vi "AuMT8852B Tester RS232 Baud Rate.vi"(5 "Baud Rate (1200)":T1(ring), 7 "Set/Get (Set)":enum16{"Set", "Get"}(ring), 8 "error in (no error)":errorcluster, 11 "VISA session":refnum<visa-resource-name>) -> (0 "error out":errorcluster, 2 "error code":i32, 3 "VISA session out":refnum<visa-resource-name>, 4 "Baud Rate Out":T1(ring))   [LabVIEW 2017]
doc: "Anritsu MT8852B Bluetooth Tester\n\nINPUTS\nSet/Get - whether the value is being sent to or retrieved from the instrument.\nBaud Rate - information to send to the instrument.\n\nOUTPUTS\nBaud Rate out - the present value in the instrument."
uses:
  <instrlib>/aumt8852B/General/Utilities/MT8850 Attribute ID.ctl
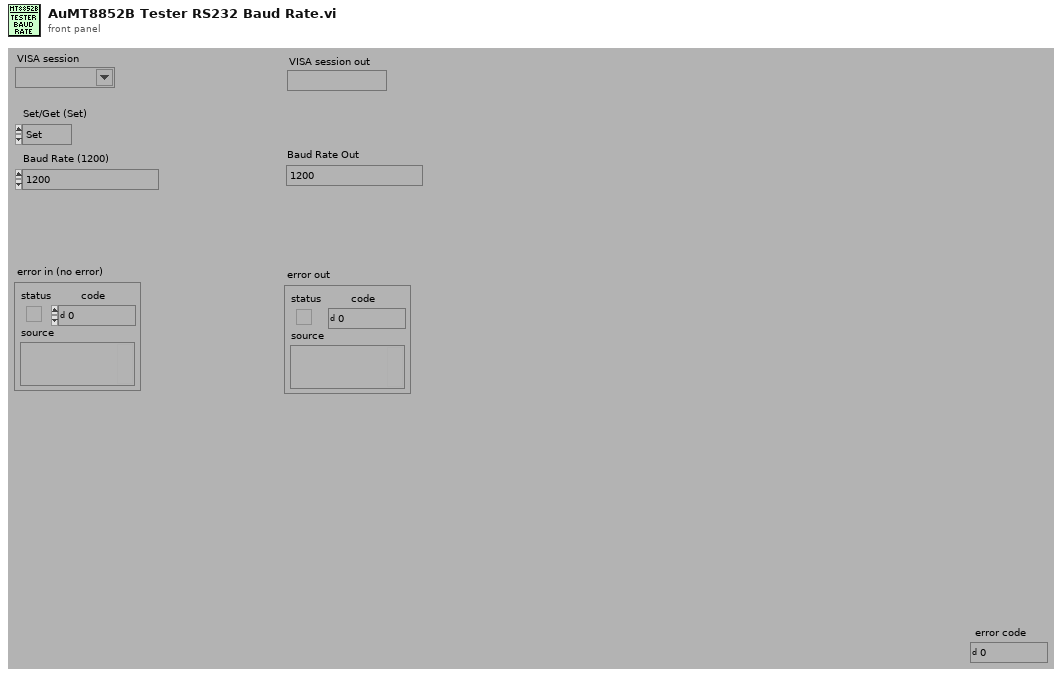
[diagram p1: front panel]
types:
  T1 = enum16{"1200", "2400", "4800", "9600", "19200", "38400", "57600"}
  T2 = typedef "MT8850 Attribute ID.ctl" = enum16{"Operation mode", "Selected script", "EUT address source", "EUT Address", "EUT HCI RS232 Baud Rate", "Tester GPIB Address", "Tester RS232 Baud Rate", "Tester Bluetooth Address", "Tester Contrast", "Tester Key Click On", "Tester Modulation Index", "Tester Poll-Null Mode", "Tester Power Range", "Tester RS232 Mode", "Beep on Illegal Entry", "Display User Text", "User Text", "Calibration TX Modulation DAC", "Calibration RX Channel", "Calibration TX Channel", "Calibration TX Power", "Calibration Use TX Table", "Inquiry Request User-friendly Name", "Inquiry Number of Responses", "Inquiry Timeout", "Script Frequency Display", "Script Loop Count", "Script Loop Continuously", "Script Loop Stop on Fail", "Link timeout", "Page timeout", "Filter bandwidth", "SCO air code", "SCO bit position", "SCO input code", "SCO input data", "SCO input sample size", "SCO loopback mode", "SCO packet type", "SCO tone generator", "Tester page scan repetition mode", "Tester follow test mode", "Tester authentication state", "Tester authentication pin code", "Tester authentication pin length"}
  T3 = typedef "Attribute Status.ctl" = enum16{"No I/O needed", "I/O needed"}
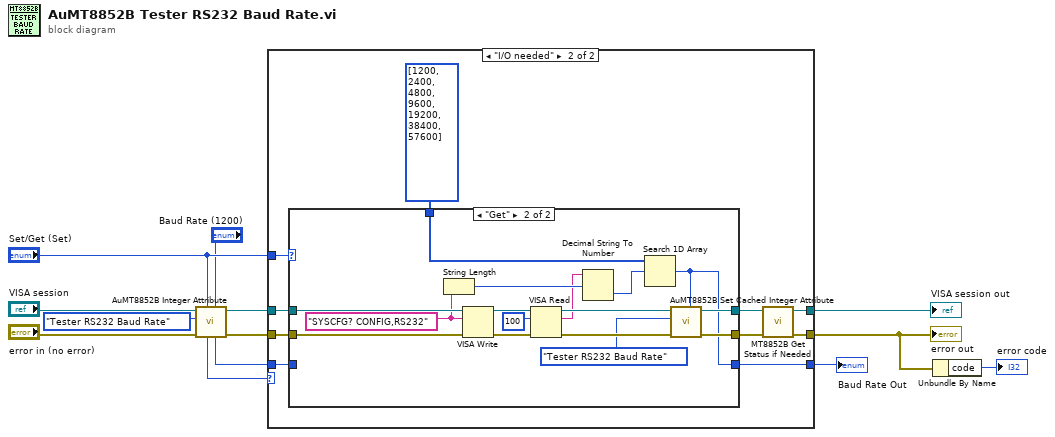
[diagram p0: block diagram]
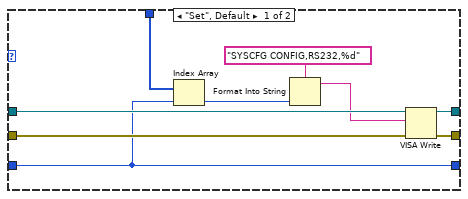
[diagram p3: hidden frame]
diagram:
  n1 = call <instrlib>:"AuMT8852B Integer Attribute.vi"("Value (0)"="Baud Rate (1200)", "Set/Get (Set)"="Set/Get (Set)", "error in (no error)"="error in (no error)", "Attribute ID"=MT8850_Attribute_ID."Tester RS232 Baud Rate", "VISA session"="VISA session") -> ("error out"=w6:errorcluster, "VISA session out"=w7:refnum<visa-resource-name>, "Value out"=w9:i32, "Status"=w4:T3)  [unwired: 3 in]
  n2 = case shown="\"I/O needed\"" w4 {
    tunnel: "Set/Get (Set)" -> [_ w26]
    tunnel: w9 -> [w16 w25]
    tunnel: [w14 w18] -> w1
    tunnel: [w15 w19] -> w8
    tunnel: w7 -> [w15 w24]
    tunnel: w6 -> [w14 w23]
    tunnel: [w16 w22] -> w3
    frame "No I/O needed", Default {
    }
    frame "I/O needed" {
      n3 = case shown="\"Get\"" w26 {
        tunnel: [w31 w44] -> w20
        tunnel: w25 -> [w33 _]
        tunnel: [w32 w45] -> w21
        tunnel: w24 -> [w35 w51]
        tunnel: w23 -> [w34 w50]
        tunnel: [w33 w43] -> w22
        tunnel: i32[] [1200, 2400, 4800, 9600, 19200, 38400, 57600] ("Array Constant") -> [w30 w38]
        frame "Set", Default {
          n4 = Index Array(array=w30, index=w33) -> (element=w28:i32)
          n5 = Format Into String(format string="SYSCFG CONFIG,RS232,%d" ("Substring"), w28) -> (resulting string=w27:string)  [unwired: 2 in, 1 out]
          n6 = VISA Write(VISA resource name=w35, write buffer=w27, error in (no error)=w34) -> (VISA resource name out=w32:refnum<visa-resource-name>, error out=w31:errorcluster)  [unwired: 1 out]
        }
        frame "Get" {
          w40 = "SYSCFG? CONFIG,RS232" ("write buffer (\"\")")
          n7 = String Length(string=w40) -> (length=w39:i32)
          n8 = VISA Write(VISA resource name=w51, write buffer=w40, error in (no error)=w50) -> (VISA resource name out=w41:refnum<visa-resource-name>, error out=w48:errorcluster)  [unwired: 1 out]
          n9 = VISA Read(VISA resource name=w41, byte count=u32 100 ("byte count (0)"), error in (no error)=w48) -> (VISA resource name out=w47:refnum<visa-resource-name>, read buffer=w36:string, error out=w46:errorcluster)  [unwired: 1 out]
          n10 = Decimal String To Number(string=w36, offset=w39) -> (number=w37:i32)  [unwired: 1 in, 1 out]
          n11 = Search 1D Array(1D array=w38, element=w37) -> (index of element=w43:i32)  [unwired: 1 in]
          n12 = call <instrlib>:"AuMT8852B Set Cached Integer Attribute.vi"("Value (0)"=w43, "error in (no error)"=w46, "Attribute ID"=MT8850_Attribute_ID."Tester RS232 Baud Rate", "VISA session"=w47) -> ("error out"=w44:errorcluster, "VISA session out"=w45:refnum<visa-resource-name>)  [unwired: 6 in]
        }
      }
      n13 = call <instrlib>:"MT8852B Get Status if Needed.vi"("error in (no error)"=w20, "VISA session"=w21) -> ("error out"=w18:errorcluster, "VISA session out"=w19:refnum<visa-resource-name>)  [unwired: 8 in]
    }
  }
  "error out" <- w1
  "VISA session out" <- w8
  "Baud Rate Out" <- w3
  n14 = Unbundle By Name(w1) -> ("code"=→"error code":i32)
